vi "InitRED.vi"(8 "error in (no error)":errorcluster, 10 "RecipeLocation":string, 11 "RecipeEditor in":refnum<class "RecipeEditor.lvclass">) -> (0 "error out":errorcluster, 3 "RecipeEditor out":refnum<class "RecipeEditor.lvclass">)   [LabVIEW 2024, in "RED Actor.lvlib" / "RecipeEditor.lvclass"]
uses:
  RecipeEditor.lvclass
  RecipeEditor.lvclass/RecipeEditor.ctl
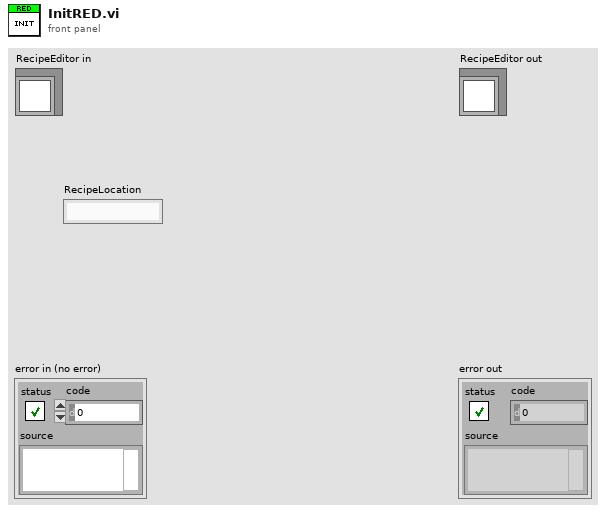
[diagram p1: front panel]
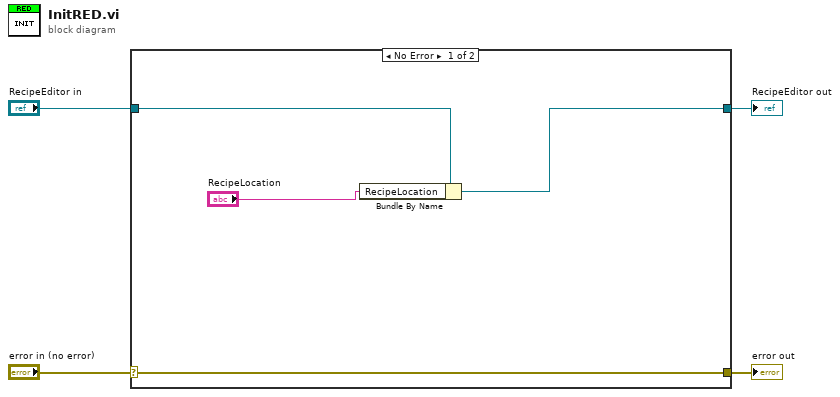
[diagram p0: block diagram]
diagram:
  n1 = case shown="No Error" "error in (no error)" {
    selector: "error in (no error)" -> [w8 w10]
    tunnel: [w8 w10] -> w3
    tunnel: [w5 w9] -> w1
    tunnel: "RecipeEditor in" -> [w6 w9]
    frame No Error {
      n2 = Bundle By Name(cluster=w6, "RecipeLocation"="RecipeLocation") -> (w5:refnum<class "RecipeEditor.lvclass">)
    }
    frame Error {
    }
  }
  "error out" <- w3
  "RecipeEditor out" <- w1
